vi "Init HT16K33.vi"(8 "error in (no error)":errorcluster, 11 "Grove I2C Matrix LED Driver in":refnum<class "Grove I2C Matrix LED Driver.lvclass">) -> (0 "error out":errorcluster, 3 "Grove I2C Matrix LED Driver out":refnum<class "Grove I2C Matrix LED Driver.lvclass">)   [LabVIEW 2020, in "CTI-Peripheral.lvlib" / "Grove I2C Matrix LED Driver.lvclass"]
uses:
  Grove I2C Matrix LED Driver.lvclass
  Grove I2C Matrix LED Driver.lvclass/Grove I2C Matrix LED Driver.ctl
  CTI/I2C Connection/I2C Connection.lvclass/I2C Connection.ctl
  CTI/Session/I2C Write Data.vi
  CTI/I2C Connection/I2C Connection.lvclass
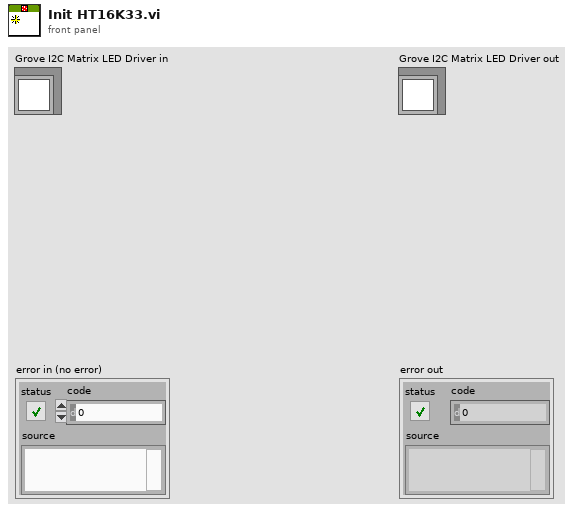
[diagram p1: front panel]
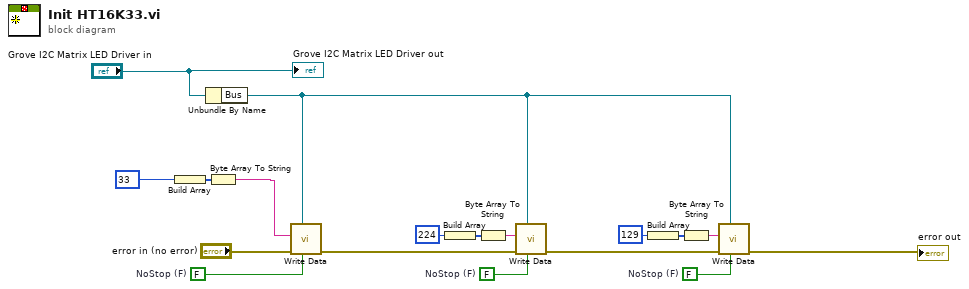
[diagram p0: block diagram]
diagram:
  w6 = FALSE  # NoStop (F)
  w10 = FALSE  # NoStop (F)
  w13 = FALSE  # NoStop (F)
  n1 = Build Array(u8 33 ("Value")) -> (w16:u8[])
  n2 = Unbundle By Name("Grove I2C Matrix LED Driver in") -> ("Bus"=w1:refnum<class "I2C Connection.lvclass">)
  n3 = Byte Array To String(unsigned byte array=w16) -> (string=w12:string)
  n4 = call "Write Data.vi"("NoStop (F)"=w13, "I2C Connection"=w1, "error in (no error)"="error in (no error)", "Data"=w12) -> ("error out"=w8:errorcluster)  [unwired: 7 in]
  n5 = Build Array(u8 224 ("Value")) -> (w15:u8[])
  n6 = Byte Array To String(unsigned byte array=w15) -> (string=w9:string)
  n7 = call "Write Data.vi"("NoStop (F)"=w10, "I2C Connection"=w1, "error in (no error)"=w8, "Data"=w9) -> ("error out"=w3:errorcluster)  [unwired: 7 in]
  n8 = Build Array(u8 129 ("Value")) -> (w4:u8[])
  n9 = Byte Array To String(unsigned byte array=w4) -> (string=w7:string)
  n10 = call "Write Data.vi"("NoStop (F)"=w6, "I2C Connection"=w1, "error in (no error)"=w3, "Data"=w7) -> ("error out"=→"error out":errorcluster)  [unwired: 7 in]
  "Grove I2C Matrix LED Driver out" <- "Grove I2C Matrix LED Driver in"
